vi "SimpleFilter2.vi"(0 "Image In":T1, 2 "Image Dst":T1, 7 "error in":errorcluster) -> (20 "Image Out":T1, 27 "error out":errorcluster)   [LabVIEW 2020]
uses:
  <vilib>/vision/Image Controls.llb/IMAQ Image.ctl
  <vilib>/vision/NI_Vision_Development_Module.lvlib
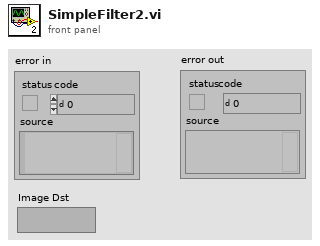
[diagram p1: front panel]
types:
  T1 = typedef "IMAQ Image.ctl" = refnum<image>
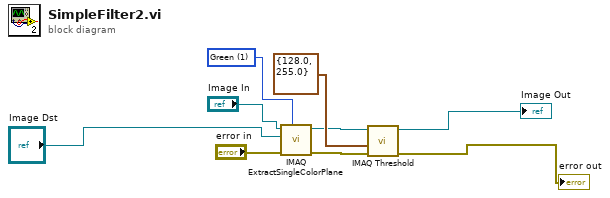
[diagram p0: block diagram]
diagram:
  w9 = 1 items=["Red", "Green", "Blue", "Hue", "Saturation", "Luminance", "Value", "Intensity"] ("Color Plane")
  n1 = call "IMAQ ExtractSingleColorPlane"("Color Plane"=w9, "error in (no error)"="error in", "Image Dst"="Image Dst", "Image Src"="Image In") -> ("error out"=w6:errorcluster, "Image Dst Out"=w2:T1)  [unwired: 6 out]
  n2 = call "IMAQ Threshold"("error in (no error)"=w6, "Range"=cluster{"Lower value":sgl, "Upper value":sgl} {"Lower value"=128.0, "Upper value"=255.0}, "Image Src"=w2) -> ("error out"=→"error out":errorcluster, "Image Dst Out"=→"Image Out":T1)  [unwired: 3 in, 4 out]
